vi "force_torque.vi"() -> ()   [LabVIEW 2013]
uses:
  <vilib>/Math Plots/3D Math Plots/3D Ribbon/3D Ribbon XCtrl/3D Ribbon.xctl
  <vilib>/Math Plots/3D Math Plots/3D Contour/3D Contour XCtrl/3D Contour.xctl
  <vilib>/Instr/_visa.llb/VISA Configure Serial Port (Instr).vi
  <vilib>/Utility/file.llb/Write To Spreadsheet File (DBL).vi
  <vilib>/Utility/file.llb/Read From Spreadsheet File (DBL).vi
  <vilib>/Utility/file.llb/Read From Spreadsheet File (string).vi
  <vilib>/Math Plots/3D Math Plots/3D Contour/3D Contour Datatype/Public/Plot Helper (Matrix).vi
  <vilib>/Math Plots/3D Math Plots/3D Ribbon/3D Ribbon Datatype/Public/Plot Helper (Matrix).vi
  <vilib>/Analysis/NI_AALPro.lvlib
  <vilib>/Math Plots/3D Math Plots/3D Ribbon/3D Ribbon Datatype/3D Ribbon Datatype.lvclass
  <vilib>/Math Plots/3D Math Plots/3D Contour/3D Contour Datatype/3D Contour Datatype.lvclass
panel:
  in  "Stop Button":bool
  in  "Tab Control":T1(tab)
  in  "off":u8=40
  in  "-мс":u32=7
  in  "end":u8=159
  in  "on":u8=52
  out "Обороты":dbl[](graph)
  in  "zero M":dbl
  in  "zero m":dbl
  in  "zeroA":dbl=16239.0
  out "ошибка":bool
  in  "Вкл модуля":bool
  in  "baud rate":u32=115200
  in  "VISA resource name":refnum<visa-resource-name>="COM7"
  out "Строка":string
  in  "Задержка":u32=5
  in  "сервосигнал":u8(knob) scale=0.0..180.0
  in  "Мотор":bool=TRUE
  in  "Тест":bool
  in  "время шага(мс)":u32=900
  in  "Очистить":bool
  out "Массив":dbl[][](array[numeric])
  out "Показания":cluster{dbl, dbl, dbl, dbl, dbl, dbl}(graph)
  out "Тяга":dbl[](graph)
  out "Момент":dbl[](graph)
  out "Ток":dbl[](graph)
  in  "Массив значений":path
  in  "Сохранить":bool
  in  "rpm k":dbl=2.0
  out "XY Graph 6":cluster{"all rows":dbl[], dbl[]}(graph)
  out "XY Graph 5":cluster{"all rows":dbl[], dbl[]}(graph)
  out "XY Graph 4":cluster{"all rows":dbl[], "all rows":dbl[]}(graph)
  out "XY Graph 3":cluster{dbl[], "all rows":dbl[]}(graph)
  in  "Tab Control 4":T2(tab)
  out "Тяга 2":dbl[](graph)
  in  "degree":i32=4
  in  "# of control points":i32=8
  in  "Применить":bool
  out "Момент 2":dbl[](graph)
  in  "Применить 2":bool
  in  "# of control points 2":i32=8
  in  "degree 2":i32=4
  out "напряжение":dbl[](graph)
  in  "Применить 3":bool
  in  "# of control points 3":i32=8
  in  "degree 3":i32=4
  out "Ток 2":dbl[](graph)
  in  "Применить 4":bool
  in  "# of control points 4":i32=8
  in  "degree 4":i32=4
  out "Обороты 2":dbl[](graph)
  in  "Применить 5":bool
  in  "# of control points 5":i32=8
  in  "degree 5":i32=4
  in  "Импорт":bool
  in  "Урезание":bool
  in  "Загрузка данных":path
  in  "Загрузка":bool
  in  "Сохранение":path
  in  "Сохранить 2":bool
  in  "spisok":bool
  in  "Y":T3(radio)
  in  "Обновить":bool
  in  "X":T3(radio)
  out "XY Graph":cluster{"all rows":dbl[], "all rows":dbl[]}[](graph)
  in  "Clear":bool
  in  "del":bool
  in  "Add":bool
  in  "Список":i32(listbox)
  in  "3d картинки":bool
  in  "Tab Control 3":enum32{"Полосы", "Поверхность"}(tab)
  out "3D Ribbon":refnum<class "3D Plot Datatype.lvclass">[](xcontrol)
  out "3D Contour":refnum<class "3D Plot Datatype.lvclass">[](xcontrol)
  in  "X 2":T3(radio)
  in  "Y 2":T3(radio)
  in  "Z":T3(radio)
  out "Ток":dbl format="%#_3g"
  in  "Вкл расчет":bool
  out "S":dbl
  out "Время мин":dbl
  out "Вт*ч":dbl
  out "Взлетная масса":dbl
  out "потребление Вт":dbl
  in  "Потребление нагрузки":dbl
  in  "Энергетическая плотность":dbl=185.0
  in  "Масса без аккумулятора грамм":dbl(slide)=1000.0 scale=600.0..5000.0
  in  "Количество моторов":u8(slide)=4 scale=2.0..16.0
  out "mAh":dbl
  out "Половина тяги":dbl
  out "XY Graph 2":cluster{"all rows":dbl[], dbl[]}(graph)
  in  "Точки по тяге":i32(listbox)
  # "0.028A 40\\52\\159    900\\7"
  # "Вт*ч/кг"
  # "Вт"
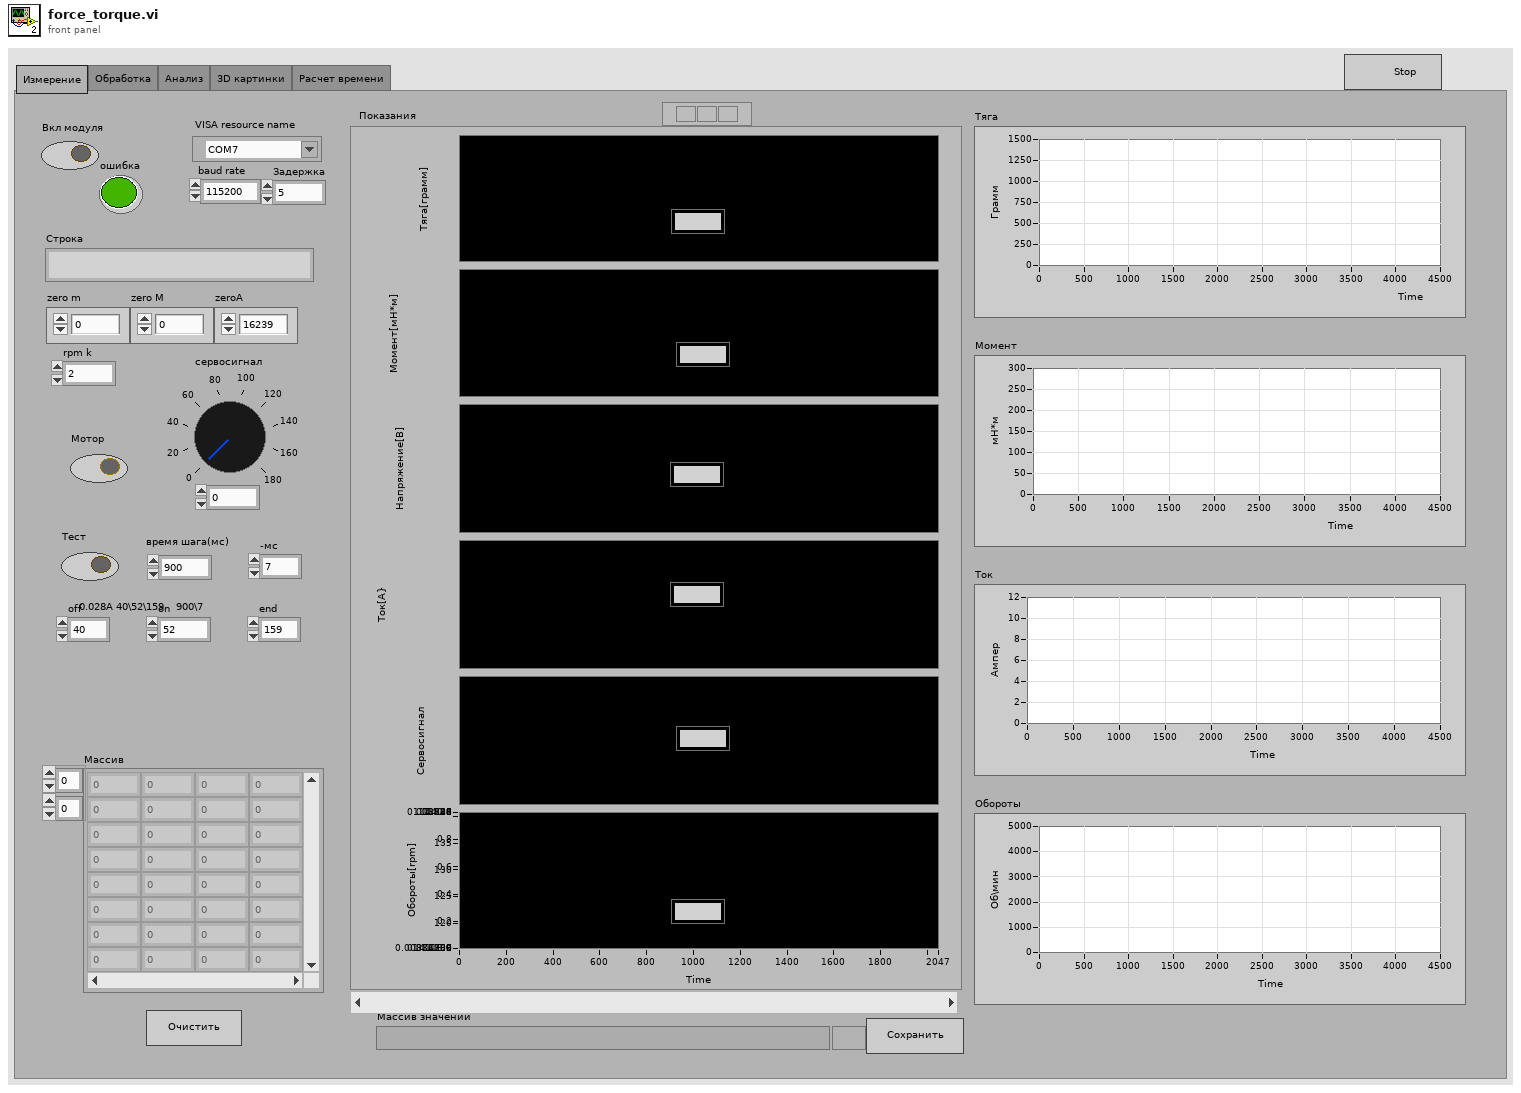
[diagram p1: front panel]
types:
  T1 = enum32{"Измерение", "Обработка", "Анализ", "3D картинки", "Расчет времени"}
  T2 = enum32{"Тяга", "Момент", "Напряжение", "Ток", "Обороты"}
  T3 = enum32{"Гр\\Вт(электро)", "Гр\\Вт(механ)", "Напряжение", "Ток", "Тяга", "Обороты", "Сервосигнал", "Мощность(Э)", "Mощность(М)", "Момент", "КПД"}
  T4 = enum32{"Гр\\Вт(электро)", "Гр\\Вт(механ)", "Напряжение", "Ток", "Тяга", "Обороты", "Сервосигнал", "Мощность(Э)", "Mощность(М)", "Момент", "КПД"}[]
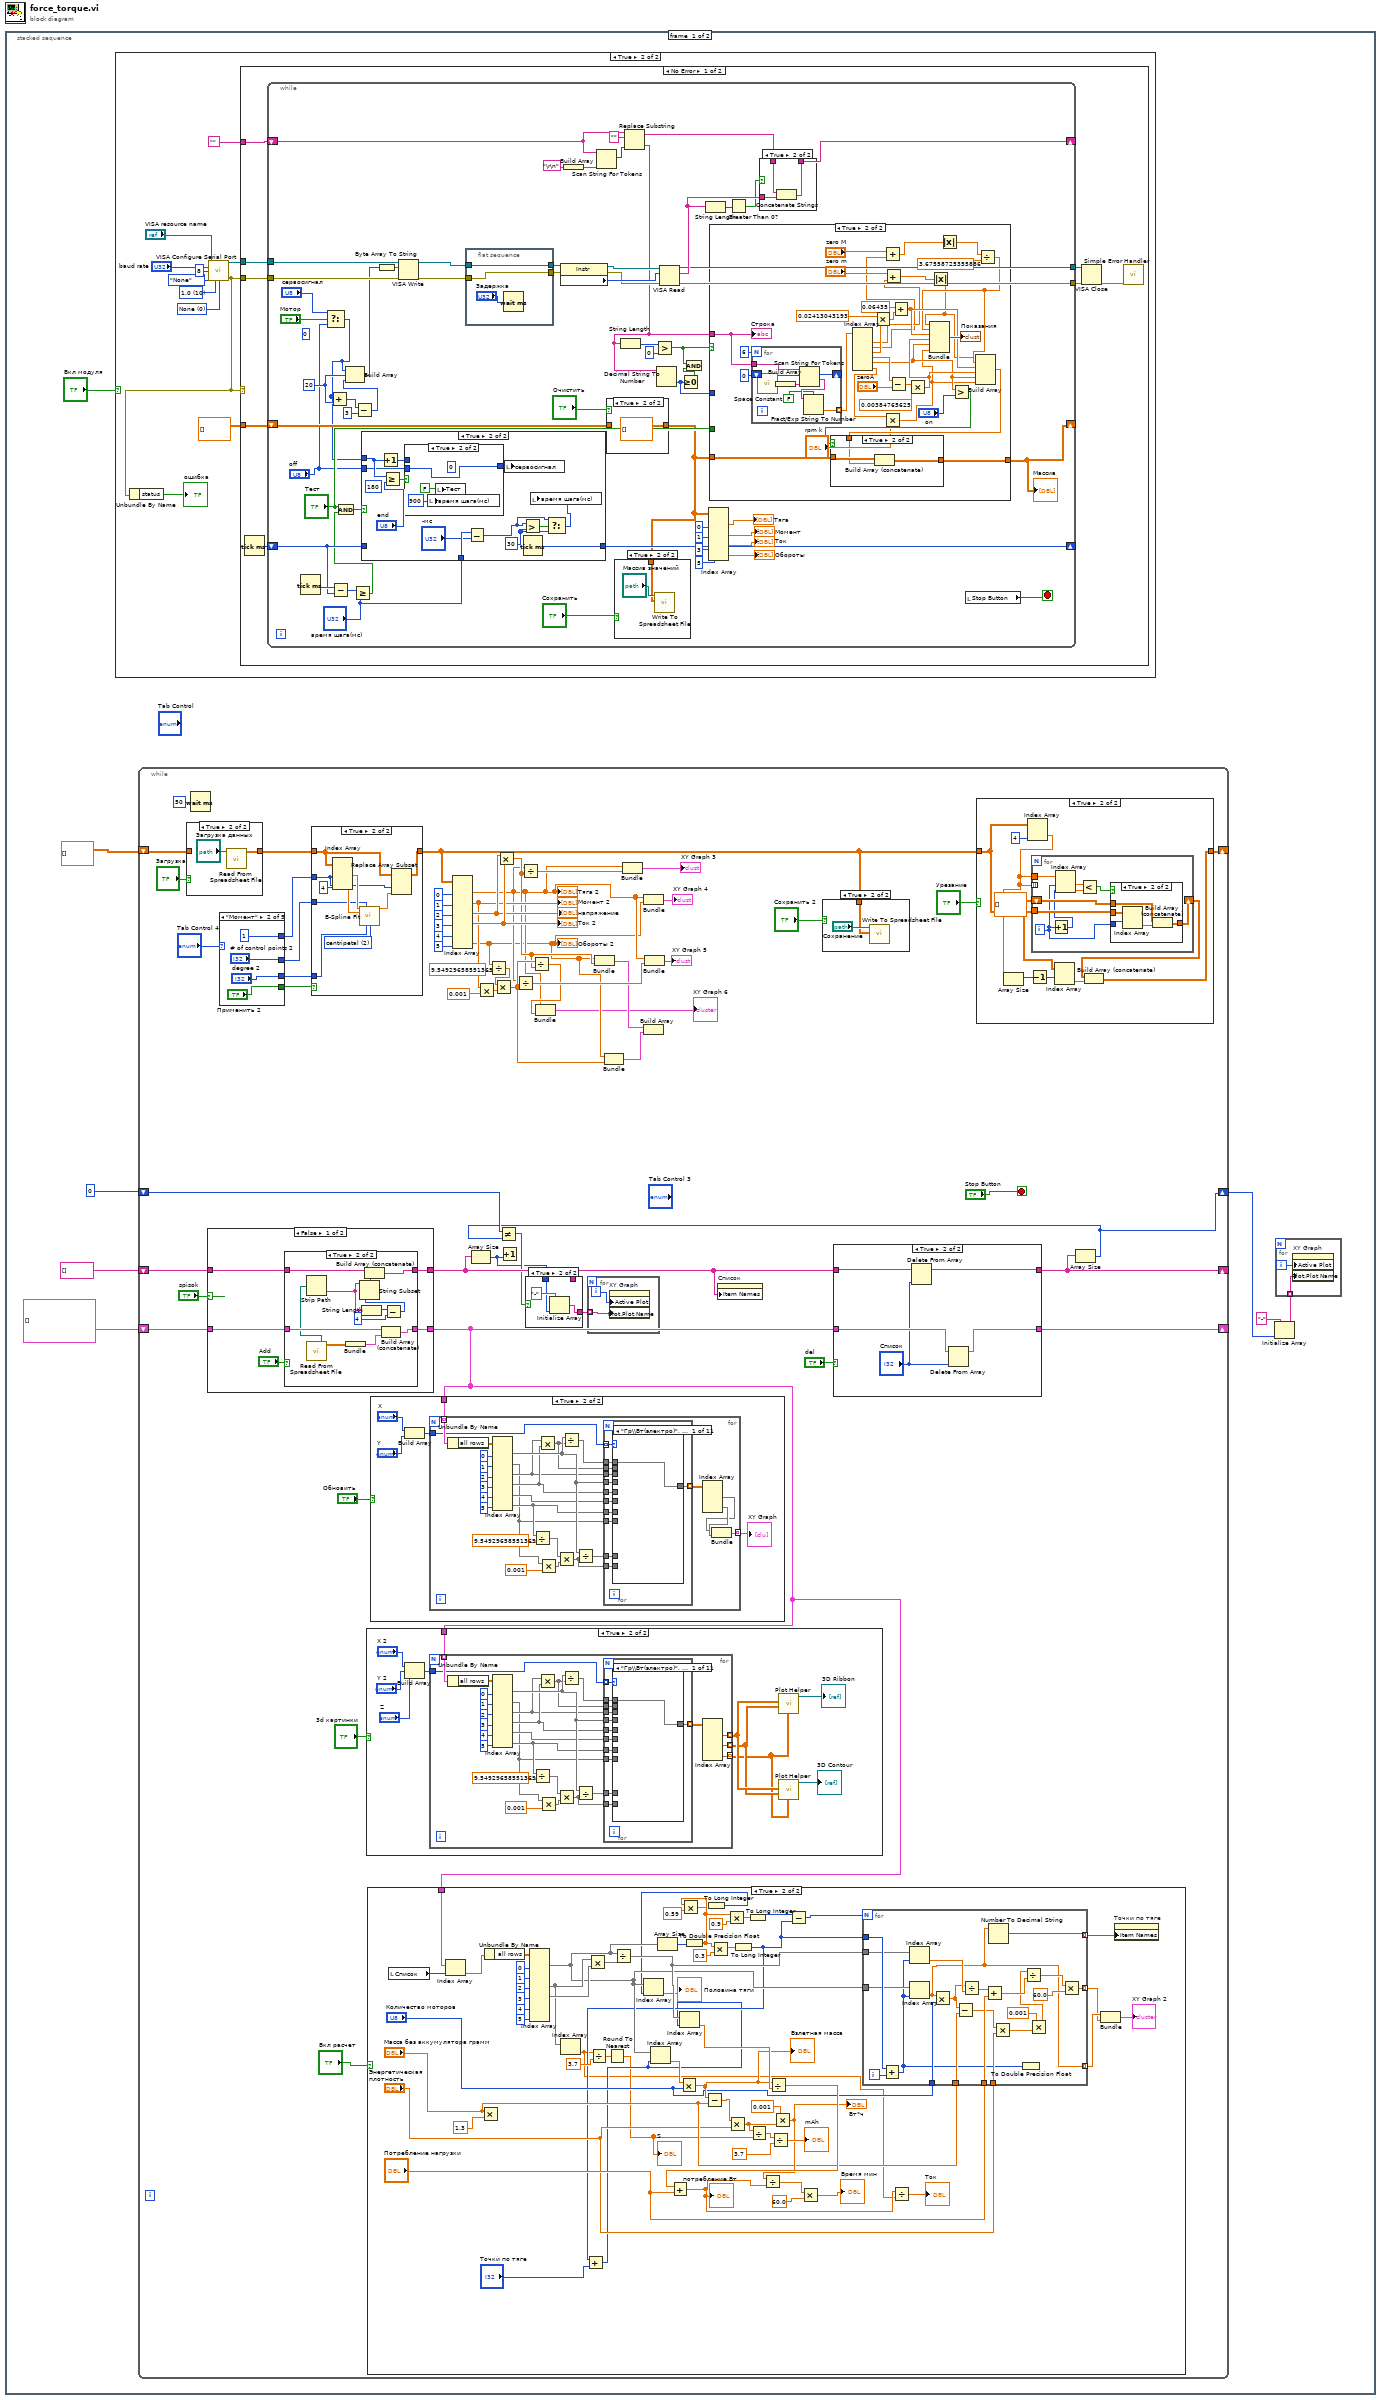
[diagram p0: block diagram]
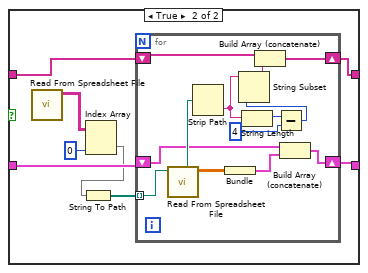
[diagram p5: hidden frame]
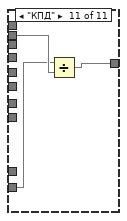
[diagram p16: hidden frame]
diagram:
  n1 = stacked-sequence {
    frame #0 {
      n2 = case shown="True" "Вкл модуля" {
        frame False {
        }
        frame True {
          w392 = u16 0 items=["None", "XON/XOFF", "RTS/CTS", "XON/XOFF & RTS/CTS", "DTR/DSR", "XON/XOFF & DTR/DSR"] ("flow control (0:none)")
          w393 = u16 10 items=["1.0"=10, "1.5"=15, "2.0"=20] ("stop bits (10: 1 bit)")
          n3 = call-poly "VISA Configure Serial Port"("VISA resource name"="VISA resource name", "baud rate (9600)"="baud rate", "data bits (8)"=u16 8, "parity (0:none)"=enum16{"None", "Odd", "Even", "Mark", "Space"}."None", "stop bits (10: 1 bit)"=w393, "flow control (0:none)"=w392) -> ("VISA resource name out"=w400:refnum<visa-resource-name>, "error out"=w396:errorcluster)  [unwired: 3 in, 5 out]
          n4 = Unbundle By Name(w396) -> ("status"=→"ошибка":bool)
          n5 = case shown="No Error" w396 {
            tunnel: w400 -> [w410 _]
            tunnel: w396 -> [w409 _]
            tunnel: "" -> [w408 _]
            tunnel: dbl[][] [] -> [w403 _]
            frame No Error {
              n6 = Tick Count (ms)() -> (millisecond timer value=w404:u32)
              n7 = while {
                tunnel: w410 -> [w453]
                tunnel: w409 -> [w452]
                shift-right: [w459] -> _
                shift-left: w408 -> [w462]
                tunnel: [w464] -> w406
                tunnel: [w426] -> w405
                shift-right: [w442] -> _
                shift-left: w404 -> [w440]
                shift-right: [w436] -> _
                shift-left: w403 -> [w434]
                stop <- w425 stop-if-true
                (unwired) u8 0 ("f")
                w451 = u8 20
                n8 = Tick Count (ms)() -> (millisecond timer value=w441:u32)
                n9 = Select(t="сервосигнал", s="Мотор", f="off") -> (s? t:f=w415:u8)
                n10 = Add(x=w415, y=w451) -> (x+y=w445:u8)
                n11 = Subtract(x=w441, y=w440) -> (x-y=w439:u32)
                n12 = Greater Or Equal?(x=w439, y="время шага(мс)") -> (x >= y?=w438:bool)
                n13 = And(x="Тест", y=w438) -> (x .and. y?=w437:bool)
                n14 = Subtract(x=w445, y=u8 3) -> (x-y=w443:u8)
                n15 = Build Array(w415, w451, w443) -> (w450:u8[])
                n16 = case shown="True" w437 {
                  tunnel: w415 -> [_ w486]
                  tunnel: [w474 w483] -> w442
                  tunnel: w440 -> [w474 _]
                  tunnel: "время шага(мс)" -> [_ w481]
                  tunnel: "off" -> [_ w475]
                  frame False {
                  }
                  frame True {
                    w478 = u32 30 ("y")
                    (unwired) u8 180
                    n17 = Increment(x=w486) -> (x+1=w484:u8)
                    n18 = Greater Or Equal?(x=w486, y="end") -> (x >= y?=w487:bool)
                    n19 = case shown="True" w487 {
                      tunnel: [w488 w490] -> w485
                      tunnel: w484 -> [w488 _]
                      tunnel: w475 -> [_ w490]
                      frame False {
                      }
                      frame True {
                        (unwired) u8 0
                        n20 = local write "время шага(мс)"(u32 900 ("время шага(мс)")) -> ()
                        n21 = local write "Тест"(FALSE) -> ()
                      }
                    }
                    n22 = Subtract(x=w481, y="-мс") -> (x-y=w477:u32)
                    n23 = local write "сервосигнал"(w485) -> ()
                    n24 = Greater?(x=w477, y=w478) -> (0:w479:bool)
                    n25 = Tick Count (ms)() -> (millisecond timer value=w483:u32)
                    n26 = Select(t=w477, s=w479, f=w478) -> (s? t:f=w476:u32)
                    n27 = local write "время шага(мс)"(w476) -> ()
                  }
                }
                n28 = Byte Array To String(unsigned byte array=w450) -> (string=w418:string)
                n29 = VISA Write(VISA resource name=w453, write buffer=w418, error in (no error)=w452) -> (VISA resource name out=w449:refnum<visa-resource-name>, error out=w447:errorcluster)  [unwired: 1 out]
                n30 = flat-sequence {
                  tunnel: w449 -> [w494]
                  tunnel: [w494] -> w448
                  tunnel: w447 -> [w493]
                  tunnel: [w493] -> w446
                  frame #0 {
                    n31 = Wait (ms)(milliseconds to wait="Задержка") -> ()  [unwired: 1 out]
                  }
                }
                n32 = property class="Instr"(reference=w448, error in=w446) -> (reference out=w468:refnum<visa-resource-name>, error out=w467:errorcluster, "Serial Settings:Number of Bytes at Serial Port"=w469:u32)
                n33 = Build Array("\r\n") -> (w423:string[])
                n34 = Scan String For Tokens(6:w423, 9:w462) -> (2:w421:i32)  [unwired: 4 in, 3 out]
                n35 = case shown="True" "Очистить" {
                  tunnel: w434 -> [w472 _]
                  tunnel: [w472 dbl[][] []] -> w419
                  frame False {
                  }
                  frame True {
                  }
                }
                n36 = case shown="True" "Сохранить" {
                  tunnel: w419 -> [_ w470]
                  frame False {
                  }
                  frame True {
                    n37 = call-poly <vilib>:"Write To Spreadsheet File.vi"("2D data"=w470, "file path (dialog if empty)"="Массив значений") -> ()  [unwired: 6 in, 1 out]
                  }
                }
                n38 = Replace Substring(2:w421, 4:"" ("substring (\"\")"), 5:w462) -> (0:w454:string, 1:w463:string)  [unwired: 1 in]
                n39 = String Length(string=w454) -> (length=w460:i32)
                n40 = Greater?(x=w460, y=0) -> (0:w455:bool)
                n41 = Decimal String To Number(string=w454) -> (number=w456:i32)  [unwired: 2 in, 1 out]
                n42 = VISA Read(VISA resource name=w468, byte count=w469, error in (no error)=w467) -> (VISA resource name out=w464:refnum<visa-resource-name>, read buffer=w465:string, error out=w426:errorcluster)  [unwired: 1 out]
                n43 = Greater Or Equal To 0?(x=w456) -> (x >= 0?=w457:bool)
                n44 = And(x=w455, y=w457) -> ()  [unwired: 1 out]
                n45 = String Length(string=w465) -> (length=w466:i32)
                n46 = Index Array(array=w419, index (col) #1=0 ("disabled index (col)"), index (col) #2=1 ("index (col)"), index (col) #3=3 ("index (col)"), index (col) #4=5 ("index (col)")) -> (element #1=→"Тяга":dbl[], element #2=→"Момент":dbl[], element #3=→"Ток":dbl[], element #4=→"Обороты":dbl[])  [unwired: 4 in]
                n47 = case shown="True" w455 {
                  tunnel: w454 -> [_ w527]
                  tunnel: w456 -> [_ _]
                  tunnel: "Тест" -> [_ _]
                  tunnel: w419 -> [w495 w525]
                  tunnel: [w495 w523] -> w436
                  frame False {
                  }
                  frame True {
                    n48 = for {
                      N: 6 -> [_]
                      tunnel: w527 -> [w540]
                      shift-right: [w538] -> _
                      shift-left: 0 -> [w537]
                      tunnel: [w535] -> w524 mode=indexing
                      n49 = call <vilib>:"Space Constant.vi"() -> ("String"=w539:string)
                      n50 = Build Array(w539) -> (w541:string[])
                      n51 = Scan String For Tokens(6:w541, 8:w537, 9:w540) -> (1:w536:string, 2:w538:i32)  [unwired: 3 in, 2 out]
                      n52 = Fract/Exp String To Number(use system decimal point (T)=FALSE, string=w536) -> (number=w535:dbl)  [unwired: 2 in, 1 out]
                    }
                    n53 = Index Array(array=w524) -> (element #1=w508:dbl, element #2=w506:dbl, element #3=w520:dbl, element #4=w517:dbl, element #5=w510:dbl, element #6=w502:dbl)  [unwired: 6 in]
                    n54 = Multiply(x=0.02413043193, y=w520) -> (x*y=w519:dbl)
                    n55 = Add(x="zero M", y=w506) -> (x+y=w499:dbl)
                    n56 = Multiply(x=w502, y="rpm k") -> (x*y=w501:dbl)
                    n57 = Add(x="zero m", y=w508) -> (x+y=w497:dbl)
                    n58 = Subtract(x=w517, y="zeroA") -> (x-y=w516:dbl)
                    n59 = Add(x=0.06435, y=w519) -> (x+y=w512:dbl)
                    n60 = Multiply(x=w516, y=0.00384765625) -> (x*y=w511:dbl)
                    n61 = Absolute Value(x=w497) -> (abs(x)=w496:dbl)
                    n62 = Absolute Value(x=w499) -> (abs(x)=w498:dbl)
                    n63 = Greater?(x=w510, y="on") -> (0:w513:bool)
                    n64 = Divide(x=w498, y=3.67558725355886) -> (x/y=w504:dbl)
                    n65 = Bundle(w496, w504, w512, w511, w510, w501) -> (→"Показания":cluster{dbl, dbl, dbl, dbl, dbl, dbl})  [unwired: 1 in]
                    n66 = Build Array(w496, w504, w512, w511, w510, w501) -> (w522:dbl[])
                    n67 = case shown="True" w513 {
                      tunnel: w525 -> [w530 w533]
                      tunnel: w522 -> [_ w532]
                      tunnel: [w530 w531] -> w523
                      frame False {
                      }
                      frame True {
                        n68 = Build Array (concatenate)(w533, w532) -> (w531:dbl[][])
                      }
                    }
                    "Строка" <- w527
                  }
                }
                "Массив" <- w436
                n69 = Greater Than 0?(x=w466) -> (x > 0?=w458:bool)
                n70 = case shown="True" w458 {
                  tunnel: w465 -> [_ w545]
                  tunnel: w463 -> [w542 w544]
                  tunnel: [w542 w543] -> w459
                  frame False {
                  }
                  frame True {
                    n71 = Concatenate Strings(w544, w545) -> (w543:string)
                  }
                }
                n72 = local read "Stop Button"() -> (w425:bool)
              }
              n73 = VISA Close(VISA resource name=w406, error in (no error)=w405) -> (error out=w407:errorcluster)
              n74 = call <vilib>:"Simple Error Handler.vi"("error in (no error)"=w407) -> ()  [unwired: 1 in, 8 out]
            }
            frame Error {
            }
          }
        }
      }
      n75 = while {
        shift-right: [w60] -> _
        shift-left: dbl[][] [] -> [w62]
        shift-right: [w21] -> _
        shift-left: cluster{dbl[][]}[] [] -> [w56]
        shift-right: [w16] -> _
        shift-left: string[] [] -> [w54]
        shift-right: [w15] -> w1
        shift-left: 0 -> [w17]
        stop <- "Stop Button" stop-if-true
        n76 = case shown="True" "Загрузка" {
          tunnel: w62 -> [w389 _]
          tunnel: [w389 w391] -> w63
          frame False {
          }
          frame True {
            n77 = call-poly <vilib>:"Read From Spreadsheet File.vi"("file path (dialog if empty)"="Загрузка данных") -> ("all rows"=w391:dbl[][])  [unwired: 6 in, 4 out]
          }
        }
        n78 = Wait (ms)(milliseconds to wait=u32 50) -> ()  [unwired: 1 out]
        n79 = case shown="False" "spisok" {
          tunnel: w56 -> [w155 w177]
          tunnel: w54 -> [w154 w178]
          tunnel: [w153 w175] -> w18
          tunnel: [w152 w176] -> w12
          frame False {
            n80 = case shown="True" "Add" {
              tunnel: w155 -> [w158 w170]
              tunnel: [w158 w169] -> w152
              tunnel: w154 -> [w157 w167]
              tunnel: [w157 w166] -> w153
              frame False {
              }
              frame True {
                n81 = call-poly <vilib>:"Read From Spreadsheet File.vi"() -> ("all rows"=w165:dbl[][], "new file path (Not A Path if cancelled)"=w168:path)  [unwired: 7 in, 3 out]
                n82 = Strip Path(path=w168) -> (name=w160:string)  [unwired: 1 out]
                n83 = Bundle("all rows"=w165) -> (w164:cluster{"all rows":dbl[][]})  [unwired: 1 in]
                n84 = String Length(string=w160) -> (length=w163:i32)
                n85 = Build Array (concatenate)(w170, w164) -> (w169:cluster{"all rows":dbl[][]}[])
                n86 = Subtract(x=w163, y=4) -> (x-y=w161:i32)
                n87 = String Subset(string=w160, length (rest)=w161) -> (substring=w159:string)  [unwired: 1 in]
                n88 = Build Array (concatenate)(w167, w159) -> (w166:string[])
              }
            }
          }
          frame True {
            n89 = call-poly <vilib>:"Read From Spreadsheet File.vi"() -> ("all rows"=w174:string[][])  [unwired: 7 in, 4 out]
            n90 = Index Array(array=w174, index (col)=0 ("disabled index (col)")) -> (element=w173:string[])  [unwired: 1 in]
            n91 = String To Path(string=w173) -> (path=w171:path[])
            n92 = for {
              shift-right: [w187] -> w175
              shift-left: w178 -> [w188]
              shift-right: [w186] -> w176
              shift-left: w177 -> [w185]
              tunnel: w171 -> [w184] mode=indexing
              n93 = call-poly <vilib>:"Read From Spreadsheet File.vi"("file path (dialog if empty)"=w184) -> ("all rows"=w190:dbl[][], "new file path (Not A Path if cancelled)"=w191:path)  [unwired: 6 in, 3 out]
              n94 = Strip Path(path=w191) -> (name=w183:string)  [unwired: 1 out]
              n95 = Bundle("all rows"=w190) -> (w189:cluster{"all rows":dbl[][]})  [unwired: 1 in]
              n96 = String Length(string=w183) -> (length=w182:i32)
              n97 = Subtract(x=w182, y=4) -> (x-y=w180:i32)
              n98 = String Subset(string=w183, length (rest)=w180) -> (substring=w179:string)  [unwired: 1 in]
              n99 = Build Array (concatenate)(w188, w179) -> (w187:string[])
              n100 = Build Array (concatenate)(w185, w189) -> (w186:cluster{"all rows":dbl[][]}[])
            }
          }
        }
        n101 = case shown="\"Момент\"" "Tab Control 4" {
          tunnel: [0 ("index (col)") 1 ("index (col)") 2 ("index (col)") 3 ("index (col)") 5 ("index (col)")] -> w48
          tunnel: ["# of control points" "# of control points 2" "# of control points 3" "# of control points 4" "# of control points 5"] -> w47
          tunnel: ["degree" "degree 2" "degree 3" "degree 4" "degree 5"] -> w46
          tunnel: ["Применить" "Применить 2" "Применить 3" "Применить 4" "Применить 5"] -> w45
          frame "Тяга", Default {
          }
          frame "Момент" {
          }
          frame "Напряжение" {
          }
          frame "Ток" {
          }
          frame "Обороты" {
          }
        }
        n102 = case shown="True" w45 {
          tunnel: w63 -> [w378 w388]
          tunnel: [w378 w387] -> w37
          tunnel: w48 -> [_ w381]
          tunnel: w47 -> [_ w380]
          tunnel: w46 -> [_ w379]
          frame False {
          }
          frame True {
            w382 = u16 2 items=["equally spaced", "chord length", "centripetal"] ("parameter selection")
            n103 = Index Array(array=w388, index (col) #1=w381, index (col) #2=4 ("index (col)")) -> (element #1=w386:dbl[], element #2=w383:dbl[])  [unwired: 2 in]
            n104 = call <vilib>:"B-Spline Fit.vi"("Y"=w386, "# of control points"=w380, "X"=w383, "degree"=w379, "parameter selection"=w382) -> ("Best BSpline Fit Y"=w385:dbl[])  [unwired: 1 in, 9 out]
            n105 = Replace Array Subset(array=w388, new element=w385, index (col)=w381) -> (w387:dbl[][])  [unwired: 1 in]
          }
        }
        n106 = case shown="True" "3d картинки" {
          tunnel: w12 -> [_ w201]
          frame False {
          }
          frame True {
            n107 = Build Array("X 2", "Y 2", "Z") -> (w199:T4)
            n108 = for {
              tunnel: w201 -> [w228] mode=indexing
              tunnel: w199 -> [w218]
              tunnel: [w204] -> w194 mode=indexing
              tunnel: [w203] -> w193 mode=indexing
              tunnel: [w202] -> w192 mode=indexing
              n109 = Unbundle By Name(w228) -> ("all rows"=w221:dbl[][])
              n110 = Index Array(array=w221, index (col) #1=0 ("disabled index (col)"), index (col) #2=1 ("index (col)"), index (col) #3=2 ("index (col)"), index (col) #4=3 ("index (col)"), index (col) #5=4 ("index (col)"), index (col) #6=5 ("index (col)")) -> (element #1=w216:dbl[], element #2=w205:dbl[], element #3=w214:dbl[], element #4=w215:dbl[], element #5=w208:dbl[], element #6=w211:dbl[])  [unwired: 6 in]
              n111 = Divide(x=w211, y=9.54929658551369) -> (x/y=w209:dbl[])
              n112 = Multiply(x=w214, y=w215) -> (x*y=w207:dbl[])
              n113 = Multiply(x=w205, y=0.001) -> (x*y=w219:dbl[])
              n114 = Multiply(x=w209, y=w219) -> (x*y=w206:dbl[])
              n115 = Divide(x=w216, y=w207) -> (x/y=w213:dbl[])
              n116 = Divide(x=w216, y=w206) -> (x/y=w212:dbl[])
              n117 = for {
                tunnel: w218 -> [w240] mode=indexing
                tunnel: [w239] -> w217 mode=indexing
                tunnel: w211 -> [w238]
                tunnel: w216 -> [w237]
                tunnel: w215 -> [w236]
                tunnel: w214 -> [w235]
                tunnel: w213 -> [w234]
                tunnel: w212 -> [w233]
                tunnel: w208 -> [w232]
                tunnel: w207 -> [w231]
                tunnel: w206 -> [w230]
                tunnel: w205 -> [w229]
                n118 = case shown="\"Гр\\\\Вт(электро)\", Default" w240 {
                  tunnel: [w241 w242 w243 w244 w245 w246 w247 w248 w249 w250 w251] -> w239
                  tunnel: w238 -> [_ _ _ _ _ w246 _ _ _ _ _]
                  tunnel: w237 -> [_ _ _ _ w245 _ _ _ _ _ _]
                  tunnel: w236 -> [_ _ _ w244 _ _ _ _ _ _ _]
                  tunnel: w235 -> [_ _ w243 _ _ _ _ _ _ _ _]
                  tunnel: w234 -> [w241 _ _ _ _ _ _ _ _ _ _]
                  tunnel: w233 -> [_ w242 _ _ _ _ _ _ _ _ _]
                  tunnel: w232 -> [_ _ _ _ _ _ w247 _ _ _ _]
                  tunnel: w231 -> [_ _ _ _ _ _ _ w248 _ _ w253]
                  tunnel: w230 -> [_ _ _ _ _ _ _ _ w249 _ w252]
                  tunnel: w229 -> [_ _ _ _ _ _ _ _ _ w250 _]
                  frame "Гр\\Вт(электро)", Default {
                  }
                  frame "Гр\\Вт(механ)" {
                  }
                  frame "Напряжение" {
                  }
                  frame "Ток" {
                  }
                  frame "Тяга" {
                  }
                  frame "Обороты" {
                  }
                  frame "Сервосигнал" {
                  }
                  frame "Мощность(Э)" {
                  }
                  frame "Mощность(М)" {
                  }
                  frame "Момент" {
                  }
                  frame "КПД" {
                    n119 = Divide(x=w252, y=w253) -> (x/y=w251:dbl[])
                  }
                }
              }
              n120 = Index Array(array=w217) -> (element #1=w204:dbl[], element #2=w203:dbl[], element #3=w202:dbl[])  [unwired: 6 in]
            }
            n121 = call-poly <vilib>:"Plot Helper.vi"("z matrix"=w192, "y matrix"=w193, "x matrix"=w194) -> ("3D Plot lvclass Array out"=→"3D Ribbon":refnum<class "3D Plot Datatype.lvclass">[])  [unwired: 3 in, 5 out]
            n122 = call-poly <vilib>:"Plot Helper.vi"("z matrix"=w192, "y matrix"=w193, "x matrix"=w194) -> ("3D Plot lvclass Array out"=→"3D Contour":refnum<class "3D Plot Datatype.lvclass">[])  [unwired: 3 in, 5 out]
          }
        }
        n123 = case shown="True" "Вкл расчет" {
          tunnel: w12 -> [_ w125]
          frame False {
          }
          frame True {
            n124 = local read "Список"() -> (w114:i32)
            n125 = Index Array(array=w125, index=w114) -> (element=w117:cluster{"all rows":dbl[][]})
            n126 = Multiply(x="Масса без аккумулятора грамм", y=1.3) -> ()  [unwired: 1 out]
            n127 = Unbundle By Name(w117) -> ("all rows"=w118:dbl[][])
            n128 = Index Array(array=w118, index (col) #1=0 ("disabled index (col)"), index (col) #2=1 ("index (col)"), index (col) #3=2 ("index (col)"), index (col) #4=3 ("index (col)"), index (col) #5=4 ("index (col)"), index (col) #6=5 ("index (col)")) -> (element #1=w78:dbl[], element #3=w113:dbl[], element #4=w116:dbl[])  [unwired: 6 in, 3 out]
            n129 = Index Array(array=w113) -> (element=w68:dbl)  [unwired: 1 in]
            n130 = Multiply(x=w113, y=w116) -> (x*y=w115:dbl[])
            n131 = Divide(x=w68, y=3.7) -> (x/y=w111:dbl)
            n132 = Round To Nearest(number=w111) -> (nearest integer value=w70:dbl)
            "S" <- w70
            n133 = Divide(x=w78, y=w115) -> (x/y=w88:dbl[])
            n134 = Array Size(array=w78) -> (size(s)=w109:i32)
            n135 = To Double Precision Float(number=w109) -> (double precision float=w83:dbl)
            n136 = Multiply(x=w83, y=0.59) -> (x*y=w82:dbl)
            n137 = To Long Integer(number=w82) -> (32bit integer=w77:i32)
            n138 = Index Array(array=w78, index=w77) -> (element=→"Половина тяги":dbl)
            n139 = Multiply(x=w83, y=0.3) -> (x*y=w108:dbl)
            n140 = Multiply(x=w83, y=0.9) -> (x*y=w91:dbl)
            n141 = To Long Integer(number=w108) -> (32bit integer=w72:i32)
            n142 = Add(x=w72, y="Точки по тяге") -> (x+y=w71:i32)
            n143 = Index Array(array=w78, index=w71) -> (element=w93:dbl)
            n144 = Multiply(x=w93, y="Количество моторов") -> (x*y=w100:dbl)
            "Взлетная масса" <- w100
            n145 = Index Array(array=w88, index=w71) -> (element=w102:dbl)
            n146 = Subtract(x=w100, y="Масса без аккумулятора грамм") -> (x-y=w106:dbl)
            n147 = Multiply(x=w106, y="Энергетическая плотность") -> (x*y=w99:dbl)
            n148 = To Long Integer(number=w91) -> (32bit integer=w90:i32)
            n149 = Divide(x=w99, y=w70) -> (x/y=w105:dbl)
            n150 = Divide(x=w100, y=w102) -> (x/y=w101:dbl)
            n151 = Add(x=w101, y="Потребление нагрузки") -> (x+y=w69:dbl)
            "потребление Вт" <- w69
            n152 = Divide(x=w105, y=3.7) -> (x/y=→"mAh":dbl)
            n153 = Multiply(x=0.001, y=w99) -> (x*y=w96:dbl)
            "Вт*ч" <- w96
            n154 = Divide(x=w96, y=w69) -> (x/y=w95:dbl)
            n155 = Subtract(x=w90, y=w72) -> (x-y=w89:i32)
            n156 = Multiply(x=w95, y=60.0) -> (x*y=→"Время мин":dbl)
            n157 = for {
              N: w89 -> [_]
              tunnel: w72 -> [w146]
              tunnel: w88 -> [w145]
              tunnel: w78 -> [w144]
              tunnel: "Количество моторов" -> [w143]
              tunnel: "Потребление нагрузки" -> [w140]
              tunnel: "Масса без аккумулятора грамм" -> [w138]
              tunnel: "Энергетическая плотность" -> [w136]
              tunnel: [w127] -> w81 mode=indexing
              tunnel: [w128] -> w80 mode=indexing
              tunnel: [w126] -> w74 mode=indexing
              i -> [w147]
              n158 = Add(x=w146, y=w147) -> (x+y=w135:i32)
              n159 = Index Array(array=w145, index=w135) -> (element=w142:dbl)
              n160 = Index Array(array=w144, index=w135) -> (element=w127:dbl)
              n161 = Multiply(x=w127, y=w143) -> (x*y=w139:dbl)
              n162 = Subtract(x=w139, y=w138) -> (x-y=w137:dbl)
              n163 = Divide(x=w139, y=w142) -> (x/y=w141:dbl)
              n164 = Add(x=w141, y=w140) -> (x+y=w132:dbl)
              n165 = Number To Decimal String(number=w127) -> (decimal integer string=w126:string)  [unwired: 1 in]
              n166 = Multiply(x=w137, y=w136) -> (x*y=w130:dbl)
              n167 = To Double Precision Float(number=w135) -> ()  [unwired: 1 out]
              n168 = Multiply(x=0.001, y=w130) -> (x*y=w129:dbl)
              n169 = Divide(x=w129, y=w132) -> (x/y=w133:dbl)
              n170 = Multiply(x=w133, y=60.0) -> (x*y=w128:dbl)
            }
            n171 = Divide(x=w69, y=w68) -> (x/y=→"Ток":dbl)
            n172 = Bundle(w81, w80) -> (→"XY Graph 2":cluster{dbl[], dbl[]})  [unwired: 1 in]
            n173 = property on="Точки по тяге" class="LstBox (strict)"("Item Names"=w74) -> ()  [unwired: 2 in, 2 out]
          }
        }
        n174 = case shown="True" "Обновить" {
          tunnel: w12 -> [_ w260]
          frame False {
          }
          frame True {
            n175 = Build Array("X", "Y") -> (w258:T4)
            n176 = for {
              tunnel: w260 -> [w287] mode=indexing
              tunnel: w258 -> [w277]
              tunnel: [w272] -> w257 mode=indexing
              n177 = Unbundle By Name(w287) -> ("all rows"=w280:dbl[][])
              n178 = Index Array(array=w280, index (col) #1=0 ("disabled index (col)"), index (col) #2=1 ("index (col)"), index (col) #3=2 ("index (col)"), index (col) #4=3 ("index (col)"), index (col) #5=4 ("index (col)"), index (col) #6=5 ("index (col)")) -> (element #1=w273:dbl[], element #2=w261:dbl[], element #3=w270:dbl[], element #4=w271:dbl[], element #5=w264:dbl[], element #6=w267:dbl[])  [unwired: 6 in]
              n179 = Divide(x=w267, y=9.54929658551369) -> (x/y=w265:dbl[])
              n180 = Multiply(x=w270, y=w271) -> (x*y=w263:dbl[])
              n181 = Multiply(x=w261, y=0.001) -> (x*y=w278:dbl[])
              n182 = Multiply(x=w265, y=w278) -> (x*y=w262:dbl[])
              n183 = Divide(x=w273, y=w263) -> (x/y=w269:dbl[])
              n184 = Divide(x=w273, y=w262) -> (x/y=w268:dbl[])
              n185 = for {
                tunnel: w277 -> [w299] mode=indexing
                tunnel: [w298] -> w274 mode=indexing
                tunnel: w267 -> [w297]
                tunnel: w273 -> [w296]
                tunnel: w271 -> [w295]
                tunnel: w270 -> [w294]
                tunnel: w269 -> [w293]
                tunnel: w268 -> [w292]
                tunnel: w264 -> [w291]
                tunnel: w263 -> [w290]
                tunnel: w262 -> [w289]
                tunnel: w261 -> [w288]
                n186 = case shown="\"Гр\\\\Вт(электро)\", Default" w299 {
                  tunnel: [w300 w301 w302 w303 w304 w305 w306 w307 w308 w309 w310] -> w298
                  tunnel: w297 -> [_ _ _ _ _ w305 _ _ _ _ _]
                  tunnel: w296 -> [_ _ _ _ w304 _ _ _ _ _ _]
                  tunnel: w295 -> [_ _ _ w303 _ _ _ _ _ _ _]
                  tunnel: w294 -> [_ _ w302 _ _ _ _ _ _ _ _]
                  tunnel: w293 -> [w300 _ _ _ _ _ _ _ _ _ _]
                  tunnel: w292 -> [_ w301 _ _ _ _ _ _ _ _ _]
                  tunnel: w291 -> [_ _ _ _ _ _ w306 _ _ _ _]
                  tunnel: w290 -> [_ _ _ _ _ _ _ w307 _ _ w311]
                  tunnel: w289 -> [_ _ _ _ _ _ _ _ w308 _ w312]
                  tunnel: w288 -> [_ _ _ _ _ _ _ _ _ w309 _]
                  frame "Гр\\Вт(электро)", Default {
                  }
                  frame "Гр\\Вт(механ)" {
                  }
                  frame "Напряжение" {
                  }
                  frame "Ток" {
                  }
                  frame "Тяга" {
                  }
                  frame "Обороты" {
                  }
                  frame "Сервосигнал" {
                  }
                  frame "Мощность(Э)" {
                  }
                  frame "Mощность(М)" {
                  }
                  frame "Момент" {
                  }
                  frame "КПД" {
                    n187 = Divide(x=w312, y=w311) -> (x/y=w310:dbl[])
                  }
                }
              }
              n188 = Index Array(array=w274) -> (element #1=w275:dbl[], element #2=w276:dbl[])  [unwired: 4 in]
              n189 = Bundle("all rows"=w275, "all rows"=w276) -> (w272:cluster{"all rows":dbl[], "all rows":dbl[]})  [unwired: 1 in]
            }
            "XY Graph" <- w257
          }
        }
        n190 = Index Array(array=w37, index (col) #1=0 ("disabled index (col)"), index (col) #2=1 ("index (col)"), index (col) #3=2 ("index (col)"), index (col) #4=3 ("index (col)"), index (col) #5=4 ("index (col)"), index (col) #6=5 ("index (col)")) -> (element #1=w30:dbl[], element #2=w39:dbl[], element #3=w43:dbl[], element #4=w44:dbl[], element #6=w27:dbl[])  [unwired: 6 in, 1 out]
        "Момент 2" <- w39
        "Тяга 2" <- w30
        "Ток 2" <- w44
        "Обороты 2" <- w27
        "напряжение" <- w43
        n191 = Array Size(array=w18) -> (size(s)=w13:i32)
        n192 = Multiply(x=w39, y=0.001) -> (x*y=w38:dbl[])
        n193 = Divide(x=w27, y=9.54929658551369) -> (x/y=w25:dbl[])
        n194 = Multiply(x=w25, y=w38) -> (x*y=w34:dbl[])
        n195 = Multiply(x=w43, y=w44) -> (x*y=w33:dbl[])
        n196 = Increment(x=w13) -> ()  [unwired: 1 out]
        n197 = Divide(x=w30, y=w34) -> (x/y=w40:dbl[])
        n198 = Divide(x=w30, y=w33) -> (x/y=w41:dbl[])
        n199 = Divide(x=w34, y=w33) -> (x/y=w31:dbl[])
        n200 = Bundle("all rows"=w30, w31) -> (→"XY Graph 6":cluster{"all rows":dbl[], dbl[]})  [unwired: 1 in]
        n201 = Bundle("all rows"=w27, w33) -> (w36:cluster{"all rows":dbl[], dbl[]})  [unwired: 1 in]
        n202 = Bundle("all rows"=w27, w34) -> (w35:cluster{"all rows":dbl[], dbl[]})  [unwired: 1 in]
        n203 = Bundle("all rows"=w30, w41) -> (→"XY Graph 3":cluster{"all rows":dbl[], dbl[]})  [unwired: 1 in]
        n204 = Bundle("all rows"=w30, "all rows"=w27) -> (→"XY Graph 4":cluster{"all rows":dbl[], "all rows":dbl[]})  [unwired: 1 in]
        n205 = Build Array(w36, w35) -> ()  [unwired: 1 out]
        n206 = Bundle("all rows"=w30, w40) -> (→"XY Graph 5":cluster{"all rows":dbl[], dbl[]})  [unwired: 1 in]
        n207 = property on="Список" class="LstBox (strict)"("Item Names"=w18) -> ()  [unwired: 2 in, 2 out]
        n208 = case shown="True" "Сохранить 2" {
          tunnel: w37 -> [_ w347]
          frame False {
          }
          frame True {
            n209 = call-poly <vilib>:"Write To Spreadsheet File.vi"("2D data"=w347, "file path (dialog if empty)"="Сохранение") -> ()  [unwired: 6 in, 1 out]
          }
        }
        n210 = case shown="True" "del" {
          tunnel: w12 -> [w336 w346]
          tunnel: [w337 w345] -> w21
          tunnel: w18 -> [w334 w344]
          tunnel: [w333 w342] -> w16
          frame False {
            n211 = case shown="True" "Clear" {
              tunnel: [w339 cluster{dbl[][]}[] []] -> w337
              tunnel: w336 -> [w339 _]
              tunnel: w334 -> [w338 _]
              tunnel: [w338 string[] []] -> w333
              frame False {
              }
              frame True {
              }
            }
          }
          frame True {
            n212 = Delete From Array(array=w344, index="Список") -> (array with subset deleted=w342:string[])  [unwired: 1 in, 1 out]
            n213 = Delete From Array(array=w346, index="Список") -> (array with subset deleted=w345:cluster{"all rows":dbl[][]}[])  [unwired: 1 in, 1 out]
          }
        }
        n214 = case shown="True" "Урезание" {
          tunnel: w37 -> [w349 w359]
          tunnel: [w350 w357] -> w60
          frame False {
            n215 = case shown="True" "Импорт" {
              tunnel: [w352 w353] -> w350
              tunnel: w349 -> [w352 _]
              frame False {
              }
              frame True {
                n216 = local read "Массив"() -> (w353:dbl[][])
              }
            }
          }
          frame True {
            n217 = Index Array(array=w359, index (col)=4) -> (element=w356:dbl[])  [unwired: 1 in]
            n218 = Array Size(array=w356) -> (size(s)=w354:i32)
            n219 = Decrement(x=w354) -> (x-1=w355:i32)
            n220 = for {
              shift-right: [w366] -> w358
              shift-left: dbl[][] [] -> [w367]
              tunnel: w356 -> [w371]
              tunnel: w359 -> [w368]
              tunnel: w356 -> [_] mode=indexing
              i -> [w363]
              n221 = Increment(x=w363) -> (x+1=w365:i32)
              n222 = Index Array(array=w371, index #1=w363, index #2=w365) -> (element #1=w369:dbl, element #2=w370:dbl)
              n223 = Less?(x=w369, y=w370) -> (x < y?=w364:bool)
              n224 = case shown="True" w364 {
                tunnel: w368 -> [_ w377]
                tunnel: w367 -> [w372 w375]
                tunnel: [w372 w374] -> w366
                tunnel: w363 -> [_ w373]
                frame False {
                }
                frame True {
                  n225 = Index Array(array=w377, index (row)=w373) -> (element=w376:dbl[])  [unwired: 1 in]
                  n226 = Build Array (concatenate)(w375, w376) -> (w374:dbl[][])
                }
              }
            }
            n227 = Index Array(array=w359, index (row)=w355) -> (element=w360:dbl[])  [unwired: 1 in]
            n228 = Build Array (concatenate)(w358, w360) -> (w357:dbl[][])
          }
        }
        n229 = Array Size(array=w16) -> (size(s)=w15:i32)
        n230 = Not Equal?(x=w17, y=w15) -> (x != y?=w14:bool)
        n231 = case shown="True" w14 {
          tunnel: [w148 w150] -> w19
          tunnel: w18 -> [w148 _]
          tunnel: w13 -> [_ w149]
          frame False {
          }
          frame True {
            n232 = Initialize Array("-", w149) -> (w150:string[])
          }
        }
        n233 = for {
          tunnel: w19 -> [w254] mode=indexing
          i -> [w255]
          n234 = property on="XY Graph" class="XYGraph (strict)"("Active Plot"=w255, "Plot.Plot Name"=w254) -> ()  [unwired: 2 in, 2 out]
        }
      }
      n235 = Initialize Array("-", w1) -> (w2:string[])
      n236 = for {
        tunnel: w2 -> [w9] mode=indexing
        i -> [w10]
        n237 = property on="XY Graph" class="XYGraph (strict)"("Active Plot"=w10, "Plot.Plot Name"=w9) -> ()  [unwired: 2 in, 2 out]
      }
    }
    frame #1 {
      n238 = local write "Stop Button"(FALSE ("Stop Button")) -> ()
    }
  }
